vi "Write value type.vi"(8 "error in (no error)":errorcluster, 10 "RndGen.Value Type":T1=enum."constant", 11 "rqcBob in":refnum<class "rqcBob.lvclass">) -> (0 "error out":errorcluster, 3 "rqcBob out":refnum<class "rqcBob.lvclass">)   [LabVIEW 2018, in "rqcBob.lvclass"]
uses:
  rqcBob.lvclass
  Shared/Shared FPGA Lib/Shared Logic/Custom Controls/rqc Random Generator.value type.ctl
  Custom Controls/rqcBob Main FPGA interface.ctl
  rqcBob.lvclass/rqcBob.ctl
  <vilib>/Utility/error.llb/Error Cluster From Error Code.vi
  <vilib>/rvi/errors/niLvFpgaAdjustHostInterfaceError.vi
  <vilib>/rvi/interface/nirviReadWriteControl/nirviReadWriteControl.xnode
  NiFpgaLv.dll
  <vilib>/rvi/interface/Simulation/niFpgaSimulationCallBeginRW.vi
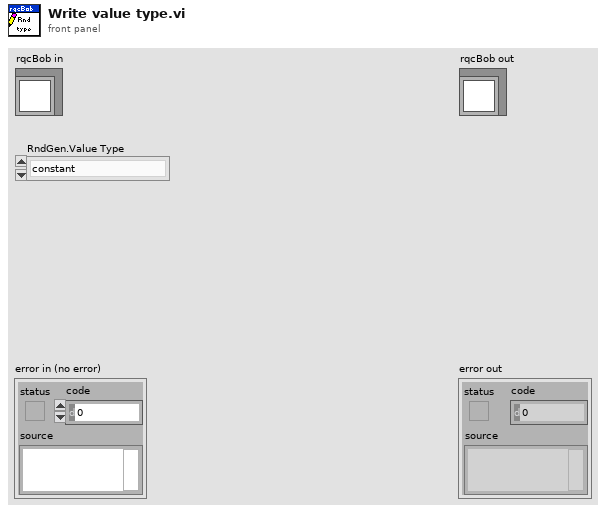
[diagram p1: front panel]
types:
  T1 = typedef "rqc Random Generator.value type.ctl" = enum16{"random value", "constant"}
  T2 = typedef "rqcBob.lvclass/rqcBob Main FPGA interface.ctl" = refnum<k20>
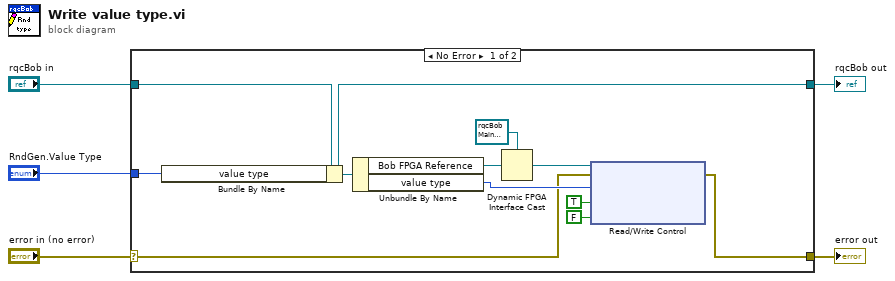
[diagram p0: block diagram]
diagram:
  n1 = case shown="No Error" "error in (no error)" {
    selector: "error in (no error)" -> [w9 w17]
    tunnel: [w8 w17] -> w4
    tunnel: [w10 w18] -> w2
    tunnel: "rqcBob in" -> [w16 w18]
    tunnel: "RndGen.Value Type" -> [w15 _]
    frame No Error {
      n2 = Bundle By Name(cluster=w16, "value type"=w15) -> (w10:refnum<class "rqcBob.lvclass">)
      n3 = Unbundle By Name(w10) -> ("Bob FPGA Reference"=w14:refnum<k20>, "value type"=w11:T1)
      n4 = Dynamic FPGA Interface Cast(Session In=T2 refnum ("Bob main FPGA interface"), Type=w14) -> (Session Out=w12:T2)
      n5 = xnode "Read/Write Control"("FPGA VI Reference In"=w12, "error in"=w9, "rndGen.value type"=w11, "rndGen.reset"=TRUE, "rndGen.reset"=FALSE) -> ("error out"=w8:errorcluster)  [unwired: 1 out]
    }
    frame Error {
    }
  }
  "error out" <- w4
  "rqcBob out" <- w2
